vi "column_width_load.vi"(8 "error in (no error)":errorcluster, 10 "configuration []":cluster{"Width":u32, "Height":u32}[](array[cluster]), 11 "listbox_reference":refnum<vi>) -> (0 "error out":errorcluster)   [LabVIEW 2015, in "lv-pagination.lvlib"]
doc: "This VI can be used to set the column width and row height of a listbox using the configuration input."
uses:
  lv-pagination.lvlib
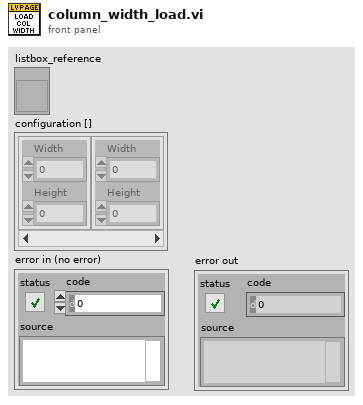
[diagram p1: front panel]
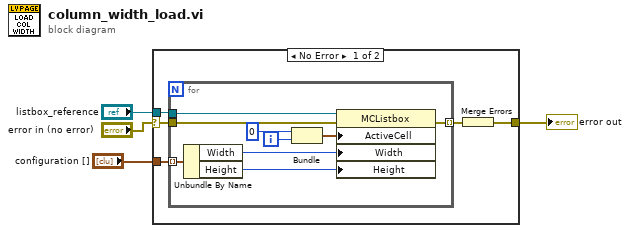
[diagram p0: block diagram]
diagram:
  n1 = case shown="No Error" "error in (no error)" {
    selector: "error in (no error)" -> [w8 w19]
    tunnel: "listbox_reference" -> [w9 _]
    tunnel: [w6 w19] -> w3
    tunnel: "configuration []" -> [w5 _]
    frame No Error {
      n2 = for {
        tunnel: w9 -> [w18]
        tunnel: [w17] -> w7 mode=indexing
        tunnel: w8 -> [w15]
        tunnel: w5 -> [w12] mode=indexing
        i -> [w14]
        n3 = Unbundle By Name(w12) -> ("Width"=w11:u32, "Height"=w10:u32)
        n4 = Bundle("Column"=0, w14) -> (w16:cluster{"Column":i32, i32})  [unwired: 1 in]
        n5 = property on="Property Node" class="MCListbox"(reference=w18, error in=w15, "ActiveCell"=w16, "Width"=w11, "Height"=w10) -> (error out=w17:errorcluster)  [unwired: 1 out]
      }
      n6 = Merge Errors(w7) -> (w6:errorcluster)
    }
    frame Error {
    }
  }
  "error out" <- w3
